vi "crc16.vi"(4 "Reflect Output? (F)":bool, 6 "Reflect Input? (F)":bool, 8 "Xor Out (0x0000)":u16 format="%04x", 9 "Poly (0x8005)":u16=32773 format="%04x", 10 "Init (0x0000)":u16 format="%04x", 11 "Data in":string) -> (3 "CRC-16":u16 format="%04x")   [LabVIEW 2020, in "wamplv.lvlib" / "HashLib.lvclass"]
doc: "Calculates a 16-bit Cyclic Redundancy Check (CRC-16) for various algorithms."
uses:
  HashLib.lvclass
  HashLib.lvclass/HashLib.ctl
panel:
  # "Data=\"123456789\"\n\nAlgorithm           Result Poly   Init   RefIn RefOut XorOut\nCRC-16/CCITT-FALSE  0x29B1 0x1021 0xFFFF false false 0x0000\nCRC-16/ARC          0xBB3D 0x8005 0x0000 true  true  0x0000\nCRC-16/AUG-CCITT    0xE5CC 0x1021 0x1D0F false false 0x0000\nCRC-16/BUYPASS      0xFEE8 0x8005 0x0000 false false 0x0000\nCRC-16/CDMA2000     0x4C06 0xC867 0xFFFF false false 0x0000\nCRC-16/DDS-110      0x9ECF 0x8005 0x800D false false 0x0000\nCRC-16/DECT-R       0x007E 0x0589 0x0000 false false 0x0001\nCRC-16/DECT-X       0x007F 0x0589 0x0000 false false 0x0000\nCRC-16/DNP          0xEA82 0x3D65 0x0000 true  true  0xFFFF\nCRC-16/EN-13757     0xC2B7 0x3D65 0x0000 false false 0xFFFF\nCRC-16/GENIBUS      0xD64E 0x1021 0xFFFF false false 0xFFFF\nCRC-16/MAXIM        0x44C2 0x8005 0x0000 true  true  0xFFFF\nCRC-16/MCRF4XX      0x6F91 0x1021 0xFFFF true  true  0x0000\nCRC-16/RIELLO       0x63D0 0x1021 0xB2AA true  true  0x0000\nCRC-16/T10-DIF      0xD0DB 0x8BB7 0x0000 false false 0x0000\nCRC-16/TELEDISK     0x0FB3 0xA097 0x0000 false false 0x0000\nCRC-16/TMS37157     0x26B1 0x1021 0x89EC true  true  0x0000\nCRC-16/USB          0xB4C8 0x8005 0xFFFF true  true  0xFFFF\nCRC-A               0xBF05 0x1021 0xC6C6 true  true  0x0000\nCRC-16/KERMIT       0x2189 0x1021 0x0000 true  true  0x0000\nCRC-16/MODBUS       0x4B37 0x8005 0xFFFF true  true  0x0000\nCRC-16/X-25         0x906E 0x1021 0xFFFF true  true  0xFFFF\nCRC-16/XMODEM       0x31C3 0x1021 0x0000 false false 0x0000\n\nSource: https://crccalc.com/"
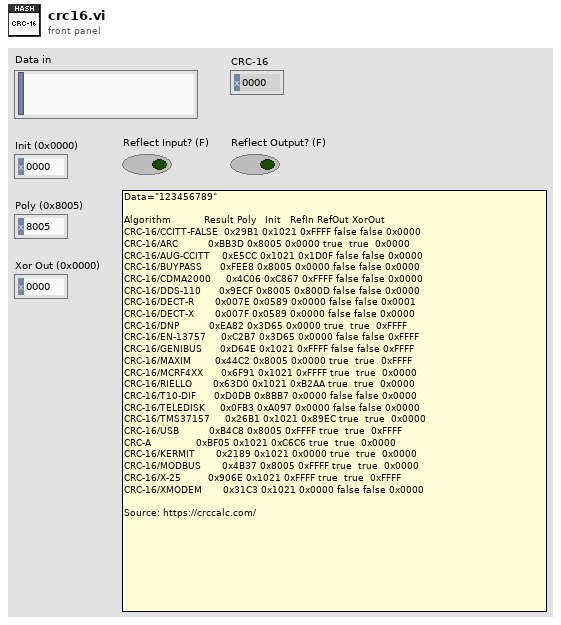
[diagram p1: front panel]
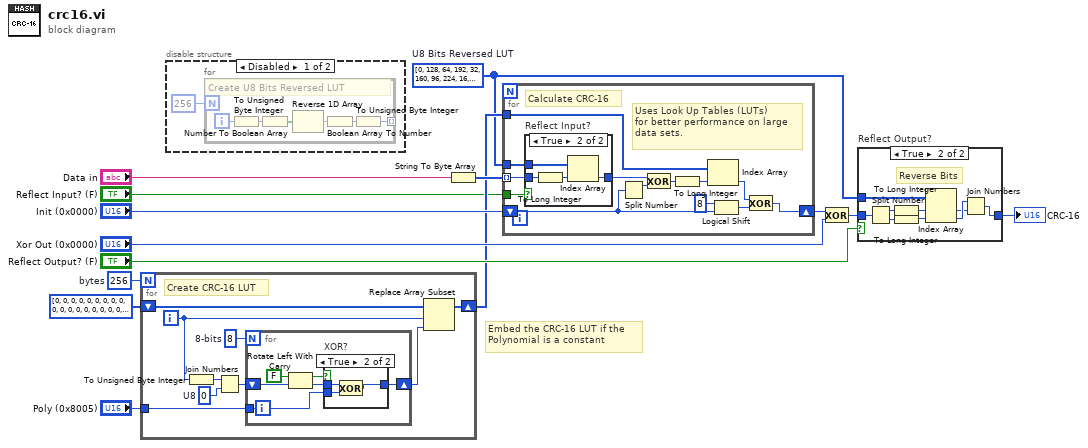
[diagram p0: block diagram]
diagram:
  w1 = u8[] [0, 128, 64, 192, 32, 160, 96, 224, 16, 144, 80, 208, 48, 176, 112, 240, 8, 136, 72, 200, 40, 168, 104, 232, 24, 152, 88, 216, 56, 184, 120, 248, 4, 132, 68, 196, 36, 164, 100, 228, 20, 148, 84, 212, 52, 180, 116, 244, 12, 140, 76, 204, 44, 172, 108, 236, 28, 156, 92, 220, 60, 188, 124, 252, 2, 130, 66, 194, 34, 162, 98, 226, 18, 146, 82, 210, 50, 178, 114, 242, 10, 138, 74, 202, 42, 170, 106, 234, 26, 154, 90, 218, 58, 186, 122, 250, 6, 134, 70, 198, 38, 166, 102, 230, 22, 150, 86, 214, 54, 182, 118, 246, 14, 142, 78, 206, 46, 174, 110, 238, 30, 158, 94, 222, 62, 190, 126, 254, 1, 129, 65, 193, 33, 161, 97, 225, 17, 145, 81, 209, 49, 177, 113, 241, 9, 137, 73, 201, 41, 169, 105, 233, 25, 153, 89, 217, 57, 185, 121, 249, 5, 133, 69, 197, 37, 165, 101, 229, 21, 149, 85, 213, 53, 181, 117, 245, 13, 141, 77, 205, 45, 173, 109, 237, 29, 157, 93, 221, 61, 189, 125, 253, 3, 131, 67, 195, 35, 163, 99, 227, 19, 147, 83, 211, 51, 179, 115, 243, 11, 139, 75, 203, 43, 171, 107, 235, 27, 155, 91, 219, 59, 187, 123, 251, 7, 135, 71, 199, 39, 167, 103, 231, 23, 151, 87, 215, 55, 183, 119, 247, 15, 143, 79, 207, 47, 175, 111, 239, 31, 159, 95, 223, 63, 191, 127, 255]  # U8 Bits Reversed LUT
  w8 = 256  # bytes
  # "Embed the CRC-16 LUT if the\nPolynomial is a constant"
  n1 = for {
    N: w8 -> [_]
    tunnel: "Poly (0x8005)" -> [w20]
    shift-right: [w16] -> w3
    shift-left: u16[] [0, 0, 0, 0, 0, 0, 0, 0, 0, 0, 0, 0, 0, 0, 0, 0, 0, 0, 0, 0, 0, 0, 0, 0, 0, 0, 0, 0, 0, 0, 0, 0, 0, 0, 0, 0, 0, 0, 0, 0, 0, 0, 0, 0, 0, 0, 0, 0, 0, 0, 0, 0, 0, 0, 0, 0, 0, 0, 0, 0, 0, 0, 0, 0, 0, 0, 0, 0, 0, 0, 0, 0, 0, 0, 0, 0, 0, 0, 0, 0, 0, 0, 0, 0, 0, 0, 0, 0, 0, 0, 0, 0, 0, 0, 0, 0, 0, 0, 0, 0, 0, 0, 0, 0, 0, 0, 0, 0, 0, 0, 0, 0, 0, 0, 0, 0, 0, 0, 0, 0, 0, 0, 0, 0, 0, 0, 0, 0, 0, 0, 0, 0, 0, 0, 0, 0, 0, 0, 0, 0, 0, 0, 0, 0, 0, 0, 0, 0, 0, 0, 0, 0, 0, 0, 0, 0, 0, 0, 0, 0, 0, 0, 0, 0, 0, 0, 0, 0, 0, 0, 0, 0, 0, 0, 0, 0, 0, 0, 0, 0, 0, 0, 0, 0, 0, 0, 0, 0, 0, 0, 0, 0, 0, 0, 0, 0, 0, 0, 0, 0, 0, 0, 0, 0, 0, 0, 0, 0, 0, 0, 0, 0, 0, 0, 0, 0, 0, 0, 0, 0, 0, 0, 0, 0, 0, 0, 0, 0, 0, 0, 0, 0, 0, 0, 0, 0, 0, 0, 0, 0, 0, 0, 0, 0, 0, 0, 0, 0, 0, 0, 0, 0, 0, 0, 0, 0] -> [w19]
    i -> [w18]
    w22 = 8  # 8-bits
    w23 = u8 0  # U8
    # "Create CRC-16 LUT"
    n2 = To Unsigned Byte Integer(number=w18) -> (unsigned 8bit integer=w15:u8)
    n3 = Join Numbers(hi=w15, lo=w23) -> ((hi.lo)=w21:u16)
    n4 = for {
      N: w22 -> [_]
      shift-right: [w25] -> w17
      shift-left: w21 -> [w29]
      tunnel: w20 -> [w26]
      n5 = Rotate Left With Carry(2:w29, 3:FALSE ("carry")) -> (0:w27:u16, 1:w24:bool)
      n6 = case "XOR?" shown="True" w24 {
        tunnel: w27 -> [w30 w33]
        tunnel: w26 -> [_ w32]
        tunnel: [w30 w31] -> w25
        frame False {
        }
        frame True {
          n7 = Exclusive Or(1:w32, 2:w33) -> (0:w31:u16)
        }
      }
    }
    n8 = Replace Array Subset(array=w19, new element=w17, index=w18) -> (w16:u16[])
  }
  n9 = disable-structure shown="Disabled" {
    frame Disabled {
      n10 = for {
        N: 256 -> [_]
        tunnel: [w35] -> _ mode=indexing
        i -> [w40]
        # "Create U8 Bits Reversed LUT"
        n11 = To Unsigned Byte Integer(number=w40) -> (unsigned 8bit integer=w39:u8)
        n12 = Number To Boolean Array(number=w39) -> (Boolean array=w38:bool[])
        n13 = Reverse 1D Array(array=w38) -> (reversed array=w37:bool[])
        n14 = Boolean Array To Number(Boolean array=w37) -> (number=w36:u32)
        n15 = To Unsigned Byte Integer(number=w36) -> (unsigned 8bit integer=w35:u8)
      }
    }
    frame Enabled {
    }
  }
  n16 = String To Byte Array(string="Data in") -> (unsigned byte array=w7:u8[])
  n17 = for {
    shift-right: [w45] -> w6
    shift-left: "Init (0x0000)" -> [w49]
    tunnel: w7 -> [w42] mode=indexing
    tunnel: w3 -> [w50]
    tunnel: "Reflect Input? (F)" -> [w41]
    tunnel: w1 -> [w44]
    # "Uses Look Up Tables (LUTs)\nfor better performance on large\ndata sets."
    # "Calculate CRC-16"
    n18 = case "Reflect Input?" shown="True" w41 {
      tunnel: w42 -> [w54 w58]
      tunnel: w44 -> [_ w56]
      tunnel: [w54 w55] -> w43
      frame False {
      }
      frame True {
        n19 = To Long Integer(number=w58) -> (32bit integer=w57:i32)
        n20 = Index Array(array=w56, index=w57) -> (element=w55:u8)
      }
    }
    n21 = Split Number(x=w49) -> (hi(x)=w53:u8)  [unwired: 1 out]
    n22 = Exclusive Or(1:w53, 2:w43) -> (0:w52:u8)
    n23 = To Long Integer(number=w52) -> (32bit integer=w51:i32)
    n24 = Index Array(array=w50, index=w51) -> (element=w46:u16)
    n25 = Logical Shift(y=i16 8, x=w49) -> (x << y=w47:u16)
    n26 = Exclusive Or(1:w47, 2:w46) -> (0:w45:u16)
  }
  n27 = Exclusive Or(1:"Xor Out (0x0000)", 2:w6) -> (0:w5:u16)
  n28 = case "Reflect Output?" shown="True" "Reflect Output? (F)" {
    tunnel: w5 -> [w59 w68]
    tunnel: [w59 w60] -> w13
    tunnel: w1 -> [_ w66]
    frame False {
    }
    frame True {
      # "Reverse Bits"
      n29 = Split Number(x=w68) -> (hi(x)=w67:u8, lo(x)=w63:u8)
      n30 = To Long Integer(number=w67) -> (32bit integer=w65:i32)
      n31 = To Long Integer(number=w63) -> (32bit integer=w64:i32)
      n32 = Index Array(array=w66, index #1=w65, index #2=w64) -> (element #1=w61:u8, element #2=w62:u8)
      n33 = Join Numbers(hi=w62, lo=w61) -> ((hi.lo)=w60:u16)
    }
  }
  "CRC-16" <- w13
